vi "Get All Attributes Priv.vi"(0 "Tree Dictionary In":variant, 5 "Unique ID":string, 11 "error in":errorcluster) -> (4 "Tree Dictionary Out":variant, 8 "Attribute Names":string[](array[string]), 10 "Attribute Values":variant[](array[variant]), 15 "error out":errorcluster)   [LabVIEW 2016, in "Tree Manager.lvclass"]
uses:
  Tree Manager.lvclass
  Typedefs/Tree.ctl
  <vilib>/Utility/error.llb/Error Cluster From Error Code.vi
  <vilib>/ErrorRing/Error Ring.xnode
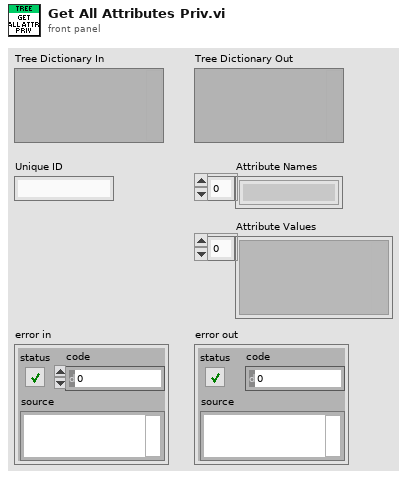
[diagram p1: front panel]
types:
  T1 = typedef "Tree Manager.lvclass/Tree.ctl" = cluster{"Unique ID":string, "Parent ID":string, "Child IDs":string[], "Data":variant, "Name":string}
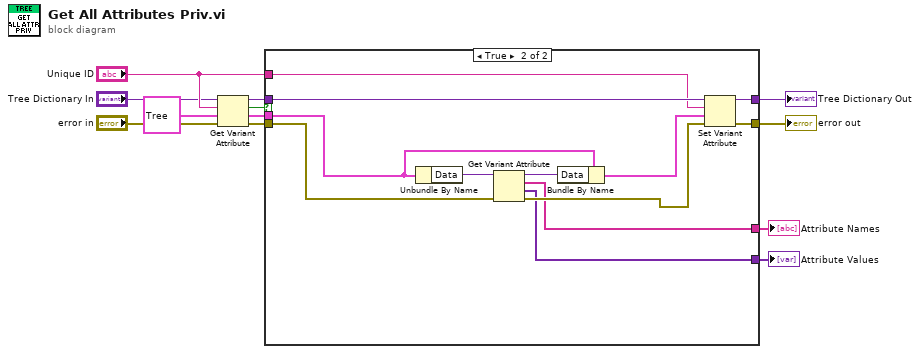
[diagram p0: block diagram]
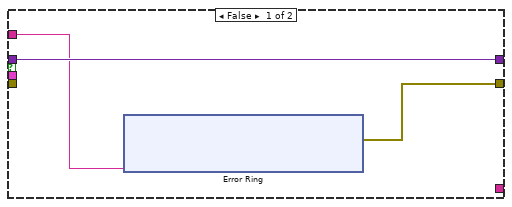
[diagram p2: hidden frame]
diagram:
  n1 = Get Variant Attribute(Variant="Tree Dictionary In", name="Unique ID", default value (empty Variant)=T1 {"Unique ID"="", "Parent ID"="", "Child IDs"=[], "Data"=variant, "Name"=""} ("Cluster of class private data"), error in="error in") -> (duplicate Variant=w9:variant, found=w10:bool, value=w11:T1, error out=w7:errorcluster)
  n2 = case shown="True" w10 {
    tunnel: [w14 w34] -> w5
    tunnel: [w15 w33] -> w6
    tunnel: w7 -> [_ w30]
    tunnel: w9 -> [w15 w32]
    tunnel: w11 -> [_ w25]
    tunnel: "Unique ID" -> [w13 w26]
    tunnel: [_ w28] -> w1
    tunnel: [_ w27] -> w2
    frame False {
      n3 = xnode "Error Ring"("parameter 0"=w13) -> ("error out"=w14:errorcluster)
    }
    frame True {
      n4 = Unbundle By Name(w25) -> ("Data"=w23:variant)
      n5 = Get Variant Attribute(Variant=w23, error in=w30) -> (duplicate Variant=w24:variant, names=w28:string[], values=w27:variant[], error out=w29:errorcluster)  [unwired: 2 in]
      n6 = Bundle By Name(cluster=w25, "Data"=w24) -> (w31:T1)
      n7 = Set Variant Attribute(Variant=w32, name=w26, value=w31, error in=w29) -> (Variant out=w33:variant, error out=w34:errorcluster)  [unwired: 1 out]
    }
  }
  "Tree Dictionary Out" <- w6
  "error out" <- w5
  "Attribute Values" <- w2
  "Attribute Names" <- w1
